vi "GetParentsRecurivly.vi"(0 "reference":refnum<class "AbstractNode.lvclass">, 5 "error in (no error)":errorcluster) -> (14 "reference out":refnum<class "AbstractNode.lvclass">, 15 "Parents":refnum<class "AbstractNode.lvclass">[](array[class]), 19 "error out":errorcluster)   [LabVIEW 2014, in "AbstractNode.lvclass"]
doc: "public Node getParent()"
uses:
  <resource>/Framework/Providers/Open_GDS/UML/AbstractNode_class/AbstractNode.lvclass
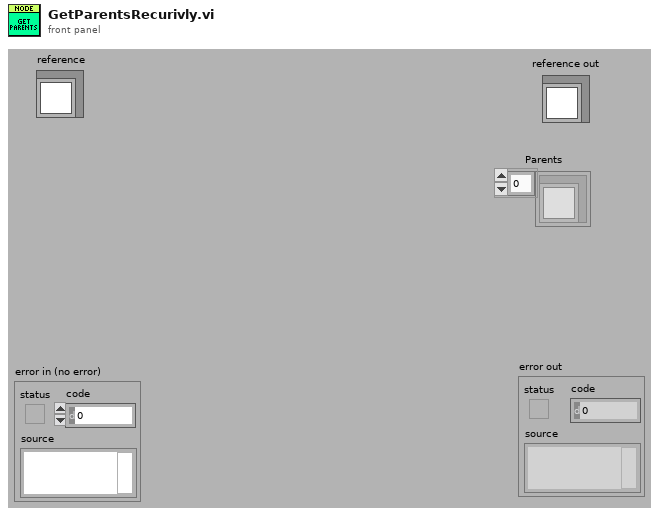
[diagram p1: front panel]
types:
  T1 = typedef "AbstractNode.lvclass/ObjectAttributes.ctl" = cluster{"parent":refnum<class "AbstractNode.lvclass">, "children":refnum<class "AbstractNode.lvclass">[], "Hidden":bool}
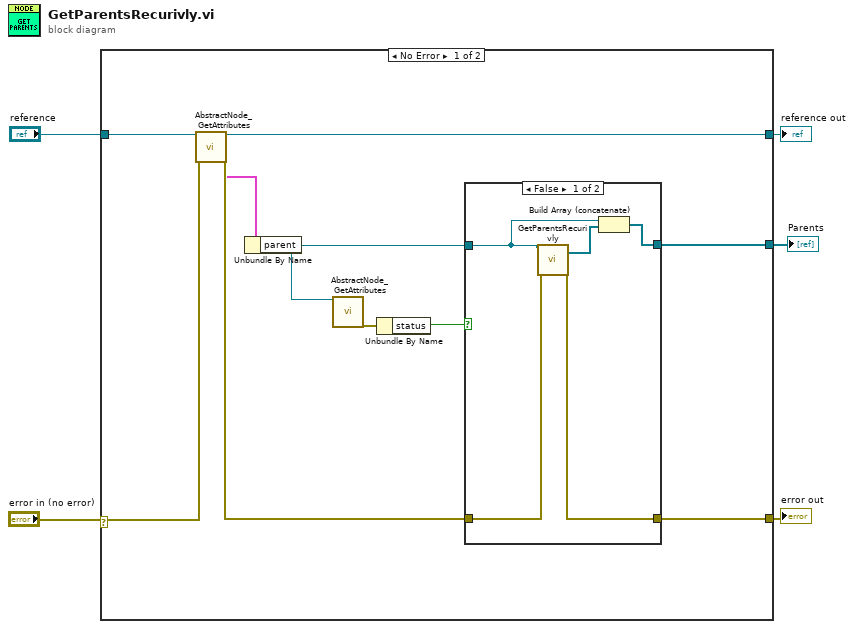
[diagram p0: block diagram]
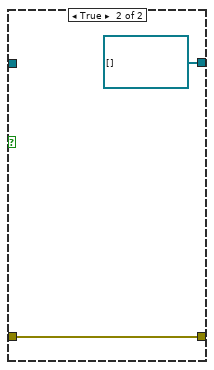
[diagram p2: hidden frame]
diagram:
  n1 = case shown="No Error" "error in (no error)" {
    selector: "error in (no error)" -> [w13 w23]
    tunnel: "reference" -> [w15 w24]
    tunnel: [w7 w23] -> w4
    tunnel: [w14 w24] -> w3
    tunnel: [w9 _] -> w1
    frame No Error {
      n2 = call <resource>:"AbstractNode_GetAttributes.vi"("reference in"=w15, "error in (no error)"=w13) -> ("reference out"=w14:refnum<class "AbstractNode.lvclass">, "Data"=w6:T1, "error out"=w8:errorcluster)  [unwired: 1 in, 14 out]
      n3 = Unbundle By Name(w6) -> ("parent"=w10:refnum<class "AbstractNode.lvclass">)
      n4 = call <resource>:"AbstractNode_GetAttributes.vi"("reference in"=w10) -> ("error out"=w12:errorcluster)  [unwired: 2 in, 16 out]
      n5 = Unbundle By Name(w12) -> ("status"=w11:bool)
      n6 = case shown="False" w11 {
        tunnel: w10 -> [w17 _]
        tunnel: [w20 refnum<class "AbstractNode.lvclass">[] []] -> w9
        tunnel: w8 -> [w19 w22]
        tunnel: [w18 w22] -> w7
        frame False {
          n7 = call-dynamic "GetParentsRecurivly.vi"("reference"=w17, "error in (no error)"=w19) -> ("Parents"=w16:refnum<class "AbstractNode.lvclass">[], "error out"=w18:errorcluster)  [unwired: 15 in, 1 out]
          n8 = Build Array (concatenate)(w17, w16) -> (w20:refnum<class "AbstractNode.lvclass">[])
        }
        frame True {
        }
      }
    }
    frame Error {
    }
  }
  "reference out" <- w3
  "error out" <- w4
  "Parents" <- w1
